vi "CCLoadDicomFile.vi"() -> ()   [LabVIEW 2013, in "main.lvlib" / "ClearCanvasLibrary.lvlib"]
uses:
  ClearCanvasLibrary.lvlib
  C:/Users/Simon/SkyDrive/LabView/2013/DM2020/DICOM/ClearCanvasNewBuild/ClearCanvas.Dicom.dll
  ClearCanvasNewBuild/ClearCanvas.Dicom.dll
panel:
  out "Save":bool
  out "Dump":string
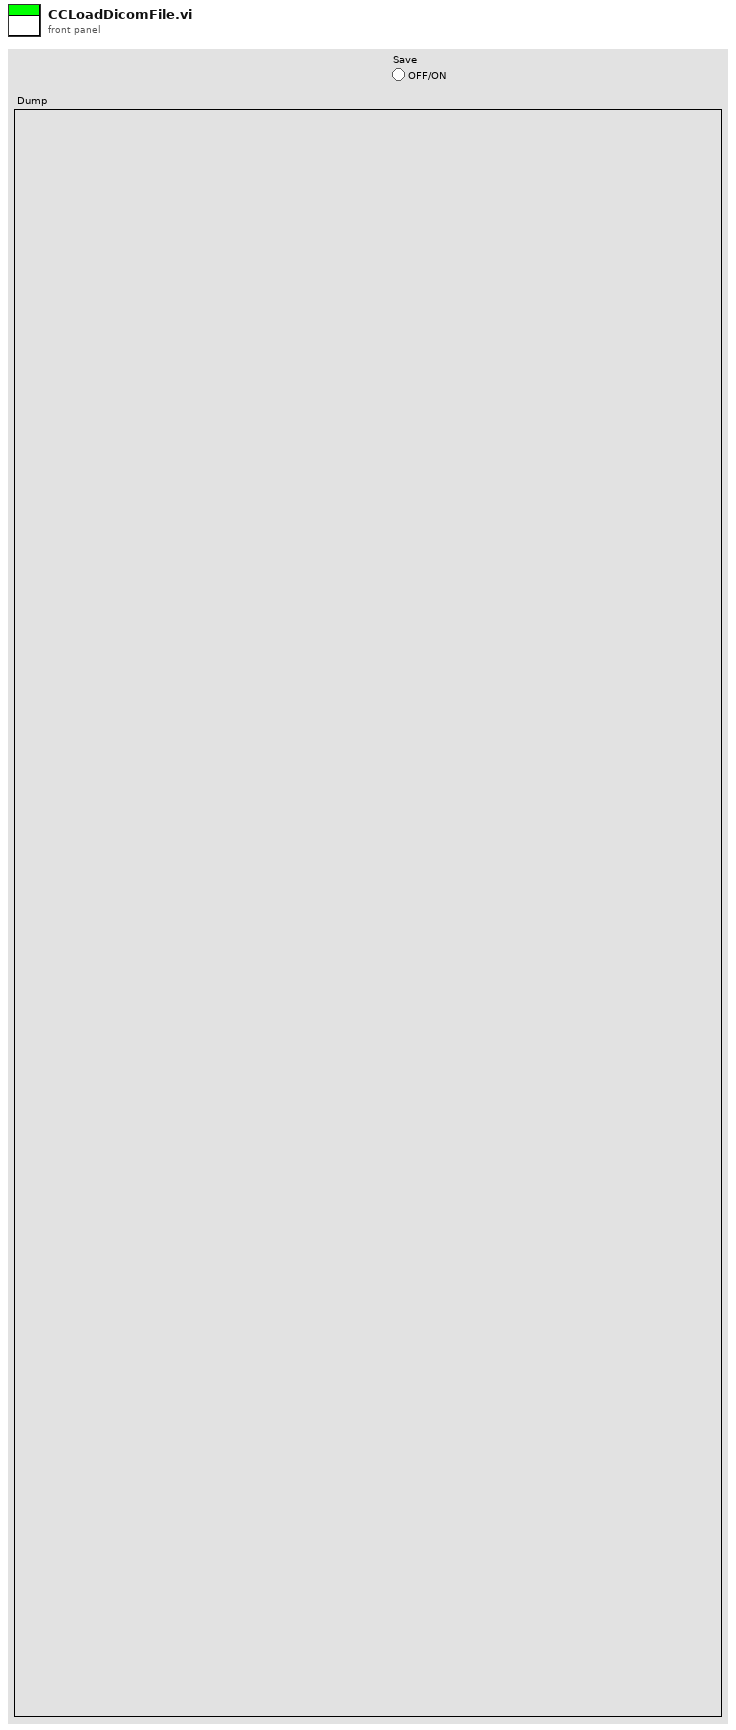
[diagram p1: front panel]
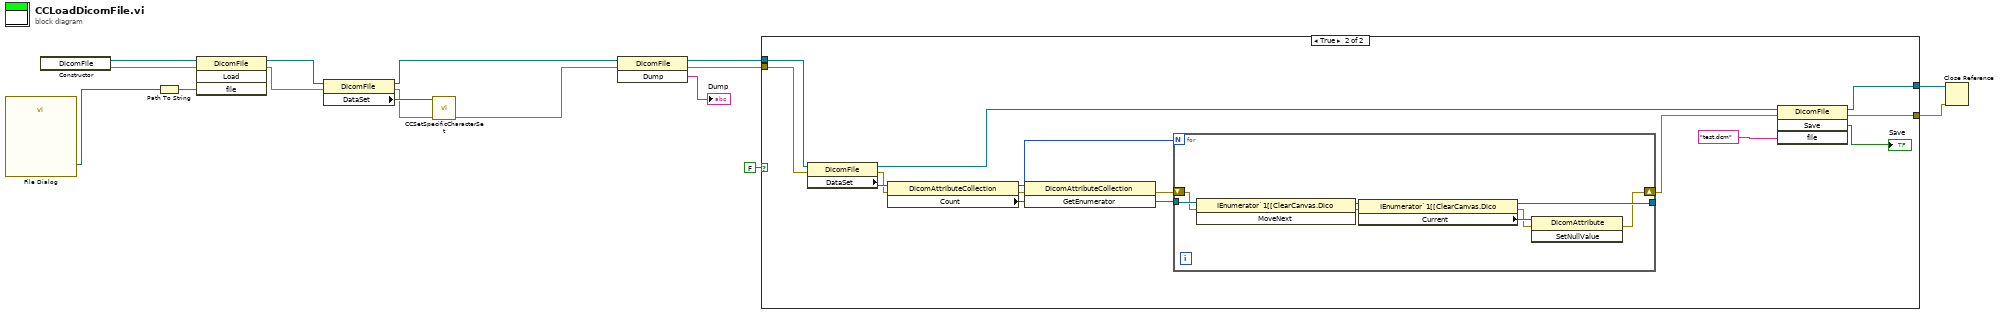
[diagram p0: block diagram]
diagram:
  n1 = call "File Dialog"() -> ("selected path"=w14:path)  [unwired: 12 in, 3 out]
  n2 = constructor class="DicomFile"() -> (reference out=w16:refnum<k24>, error out=w4:errorcluster)  [unwired: 3 in, 1 out]
  n3 = Path To String(path=w14) -> (string=w13:string)
  n4 = invoke class="DicomFile" method="Load"(reference=w16, error in=w4, "file"=w13) -> (reference out=w7:refnum<k24>, error out=w3:errorcluster)  [unwired: 1 in, 2 out]
  n5 = property class="DicomFile"(reference=w7, error in=w3) -> (reference out=w1:refnum<k24>, error out=w2:errorcluster, "DataSet"=w6:refnum<k24>)
  n6 = call "CCSetSpecificCharacterSet.vi"("error in (no error)"=w2, ".NET Refnum in"=w6) -> ("error out"=w5:errorcluster)  [unwired: 8 in, 1 out]
  n7 = invoke class="DicomFile" method="Dump"(reference=w1, error in=w5) -> (reference out=w11:refnum<k24>, error out=w12:errorcluster, "Dump"=→"Dump":string)  [unwired: 1 in]
  n8 = case shown="True" FALSE {
    tunnel: w12 -> [w18 w23]
    tunnel: w11 -> [w17 w22]
    tunnel: [w18 w21] -> w10
    tunnel: [w17 w20] -> w9
    frame False {
    }
    frame True {
      n9 = property class="DicomFile"(reference=w22, error in=w23) -> (reference out=w26:refnum<k24>, error out=w29:errorcluster, "DataSet"=w33:refnum<k24>)
      n10 = property class="DicomAttributeCollection"(reference=w33, error in=w29) -> (reference out=w32:refnum<k24>, error out=w28:errorcluster, "Count"=w31:i32)
      n11 = invoke class="DicomAttributeCollection" method="GetEnumerator"(reference=w32, error in=w28) -> (error out=w27:errorcluster, "GetEnumerator"=w30:refnum<k24>)  [unwired: 1 in, 1 out]
      n12 = for {
        N: w31 -> [_]
        tunnel: w30 -> [w41]
        tunnel: [w38] -> _
        shift-right: [w34] -> w25
        shift-left: w27 -> [w37]
        n13 = invoke class="IEnumerator`1[[ClearCanvas.Dico" method="MoveNext"(reference=w41, error in=w37) -> (reference out=w40:refnum<k24>, error out=w36:errorcluster)  [unwired: 1 in, 1 out]
        n14 = property class="IEnumerator`1[[ClearCanvas.Dico"(reference=w40, error in=w36) -> (reference out=w38:refnum<k24>, error out=w35:errorcluster, "Current"=w39:refnum<k24>)
        n15 = invoke class="DicomAttribute" method="SetNullValue"(reference=w39, error in=w35) -> (error out=w34:errorcluster)  [unwired: 1 in, 2 out]
      }
      n16 = invoke class="DicomFile" method="Save"(reference=w26, error in=w25, "file"="test.dcm") -> (reference out=w20:refnum<k24>, error out=w21:errorcluster, "Save"=→"Save":bool)  [unwired: 1 in, 1 out]
    }
  }
  n17 = Close Reference(reference=w9, error in (no error)=w10) -> ()  [unwired: 1 out]
